vi "Set CC Frame Type.vi"(8 "error in":errorcluster, 10 "CC Frame Type":enum8{"Data", "Remote", "Error", "Overload"}(ring), 11 "CANopen Message in":refnum<class "CANopen Message.lvclass">) -> (0 "error out":errorcluster, 3 "CANopen Message out":refnum<class "CANopen Message.lvclass">)   [LabVIEW 2020, in "CANopen.lvlib" / "CANopen Message.lvclass"]
uses:
  CANopen Message.lvclass
  CANopen Message.lvclass/CANopen Message.ctl
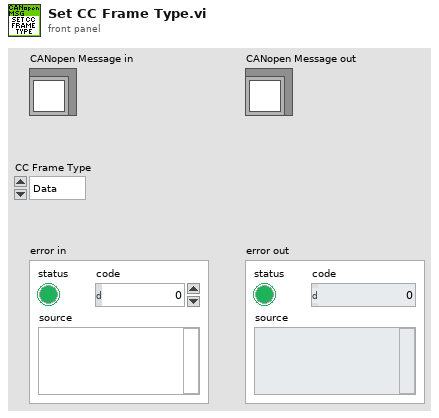
[diagram p1: front panel]
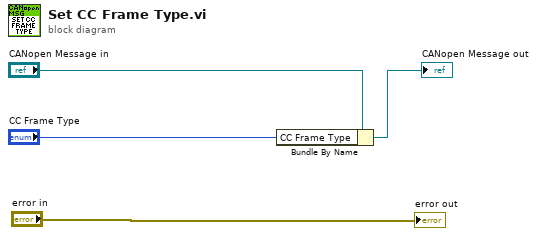
[diagram p0: block diagram]
diagram:
  n1 = Bundle By Name(cluster="CANopen Message in", "CC Frame Type"="CC Frame Type") -> (→"CANopen Message out":refnum<class "CANopen Message.lvclass">)
  "error out" <- "error in"
